vi "HiSPARCIII.vi"(6 "Files in":T1, 8 "Status/Errors in":refnum<vi>, 9 "Mode in":T2={"Mode"=enum."Dialog", "Expert?"=FALSE, "Dialog?"=FALSE}, 10 "Control Parameters [] in":T3[](array[typedef]) {"Aux Byte Value" format="%02x"; "Max Real Value" format="%#_6e"; "Min Real Value" format="%#_6e"; "dReal/dByte" format="%#_6e"; "Byte Value" format="%02x"; "Identifier" format="%02x"}) -> (0 "Status/Errors out":refnum<vi>, 1 "Mode out":T2={"Mode"=enum."Dialog", "Expert?"=FALSE, "Dialog?"=FALSE}, 2 "Control Parameters [] out":T3[](array[typedef]) {"Aux Byte Value" format="%02x"; "Max Real Value" format="%#_6e"; "Min Real Value" format="%#_6e"; "dReal/dByte" format="%#_6e"; "Byte Value" format="%02x"; "Identifier" format="%02x"}, 4 "Files out":T1)   [LabVIEW 2010]
uses:
  Controls/Control_Parameters.ctl
  Controls/Master.ctl
  Controls/Mode.ctl
  Controls/Files.ctl
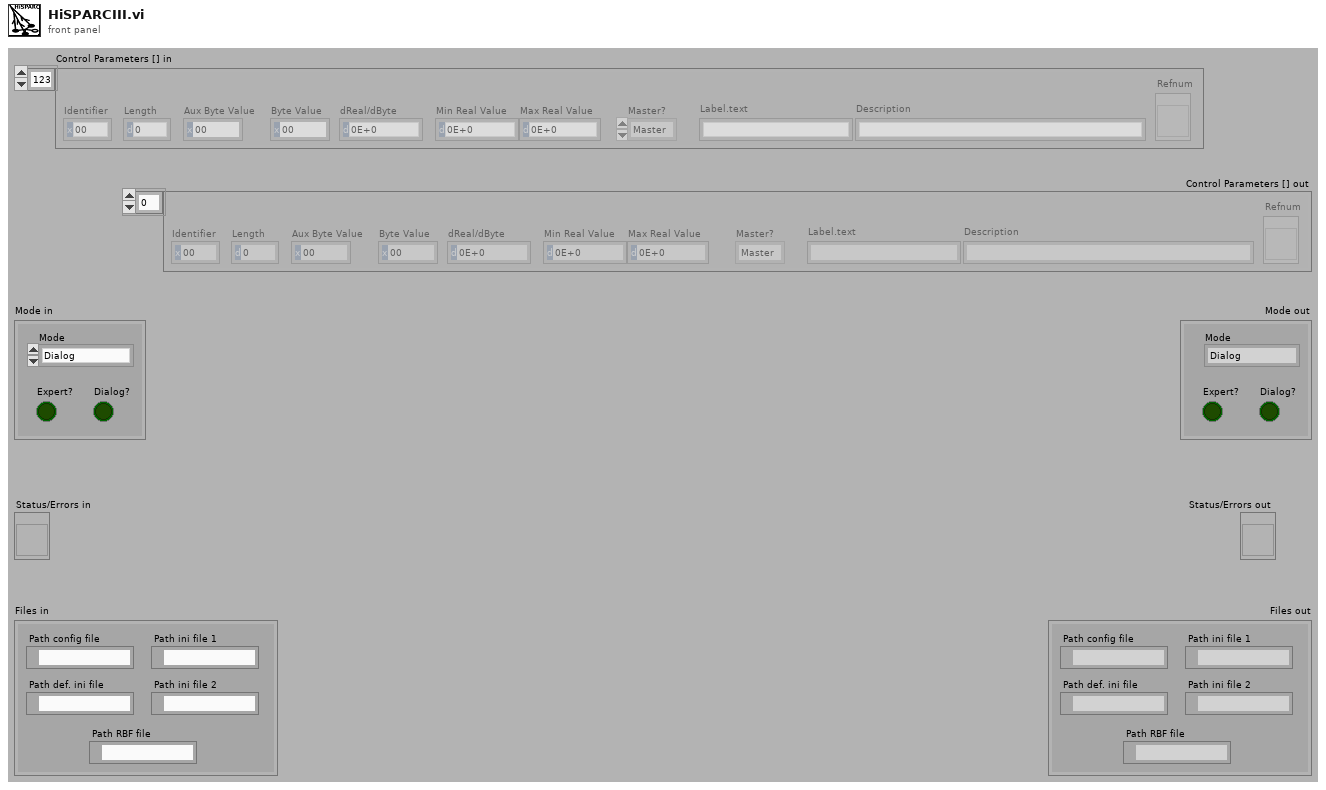
[diagram p1: front panel]
types:
  T1 = typedef "Files.ctl" = cluster{"Path config file":path, "Path def. ini file":path, "Path ini file 1":path, "Path ini file 2":path, "Path RBF file":path}
  T2 = typedef "Mode.ctl" = cluster{"Mode":enum8{"Stop", "Dialog", "Hisparc II", "Hisparc II DAQ", "Alignment"}, "Expert?":bool, "Dialog?":bool}
  T3 = typedef "Control_Parameters.ctl" = cluster{"Identifier":u8, "Length":u16, "Byte Value":u32, "dReal/dByte":dbl, "Min Real Value":dbl, "Max Real Value":dbl, "Master?":T4, "Label.text":string, "Description":string, "Refnum":refnum<vi>, "Aux Byte Value":u32}
  T4 = typedef "Master.ctl" = enum16{"Master", "Slave", "General"}
  T5 = enum8{"Stop", "Dialog", "Hisparc II", "Hisparc II DAQ", "Alignment"}
  T6 = typedef "Parameters.ctl" = cluster{"Mode":T2, "Stop loop":T7, "Send message":T8, "Write settings":T10, "Read bytes":T12, "Settings state":T13, "Button refs":T14, "Process messages":T15, "Data storage":T17, "Update screen":T22, "Alignment parameters":refnum<vi>, "Timer parameters":refnum<vi>, "Files":T1, "Status_id":refnum<vi>, "Time difference":refnum<vi>, "Satellites":refnum<vi>, "Calibration":T23, "Page Statistics 2":refnum<vi>, "Page Statistics":refnum<vi>}
  T7 = typedef "Stop_Loop.ctl" = cluster{"Settings changed?":bool, "Stop?":refnum<vi>}
  T8 = typedef "Send_Message.ctl" = cluster{"Send mode":T9, "Set parameter list":u8, "Get parameter list":u8, "Reset device":u8, "Length set settings message":i32, "Reset buttons?":bool, "Reset Master?":T4}
  T9 = typedef "Send_Message_Mode.ctl" = enum16{"Get parameters", "Set parameters", "From front panel", "From parameters", "Reset device", "Alignment"}
  T10 = typedef "Write_Settings.ctl" = cluster{"Options":T11}
  T11 = typedef "Write_Settings_Options.ctl" = enum16{"File 1", "File 2", "Alignment", "Reset"}
  T12 = typedef "Read_Bytes.ctl" = cluster{"Max bytes read":u32, "Max bytes reached?":bool}
  T13 = typedef "Settings_State.ctl" = cluster{"MAS locked?":refnum<vi>, "SLV locked?":refnum<vi>}
  T14 = typedef "Button_Refs.ctl" = cluster{"Stop program":refnum<vi>, "Save settings":refnum<vi>, "DAQ mode":refnum<vi>, "Reset settings":refnum<vi>, "Apply settings":refnum<vi>, "Reset MAS":refnum<vi>, "Reset SLV":refnum<vi>, "Local DBase?":refnum<vi>, "Last value DBase":bool, "Database":refnum<vi>, "Calibration":refnum<vi>, "Save settings 2":refnum<vi>}
  T15 = typedef "Process_Messages.ctl" = cluster{"Process message mode":T16, "Slave data?":bool, "Length get settings message":i32, "Delta time":dbl, "Data_Filter":cluster{"Filter_Data":bool, "Use_Thresh":bool, "Reduce data?":bool}, "Time_difference_stack":u64[], "Starting sec":u64, "Ending sec":u64, "Ending sec 2":u64, "MAS_Page_Thresh":refnum<vi>, "SLV_Page_Thresh":refnum<vi>, "Database":refnum<vi>}
  T16 = typedef "Process_Message_Mode.ctl" = enum16{"Error", "Measurement data", "Comparator data", "One Second"}
  T17 = typedef "Data_Storage.ctl" = cluster{"DB connection":T18, "Data storage condition":T20, "Detector number":u16, "# Messages to send":i32, "Database":refnum<vi>, "Password":string, "Last error message":cluster{"Last error message time stamp":T21, "Last error log":string, "Last error message":string}, "Status_id":refnum<vi>, "Hardware":enum8{"None", "HiSPARC I", "HiSPARC II", "HiSPARC III", "Unknown"}}
  T18 = typedef "DB_Connection.ctl" = cluster{"connection reference":T19, "Connected?":refnum<vi>, "ODBC Name":string}
  T19 = typedef "Conn ObjectReference.ctl" = refnum<k1>
  T20 = typedef "Data_Storage_Condition.ctl" = cluster{"Database?":bool}
  T21 = typedef "GPS_Timestamp.ctl" = cluster{"Seconds":u8, "Minutes":u8, "Hours":u8, "Day":u8, "Month":u8, "Year":u16}
  T22 = typedef "Update_Screen.ctl" = cluster{"Detector number":u16, "Hardware":enum8{"None", "HiSPARC I", "HiSPARC II", "HiSPARC III", "Unknown"}}
  T23 = typedef "Page_Calibration.ctl" = cluster{"GEN_Page_Calibrate":refnum<vi>, "MAS_Page_Gain":refnum<vi>, "MAS_Page_Offset":refnum<vi>, "SLV_Page_Gain":refnum<vi>, "SLV_Page_Offset":refnum<vi>, "MAS_Page_Common":refnum<vi>, "SLV_Page_Common":refnum<vi>}
  T24 = typedef "Devices.ctl" = cluster{"Master":refnum<vi>, "Slave":refnum<vi>}
  T25 = typedef "Queues.ctl" = cluster{"MAS":cluster{"Bytes":refnum<queue>, "Settings":refnum<queue>, "Errors":refnum<queue>, "Meas. data":refnum<queue>, "One Second":refnum<queue>, "Comp. data":refnum<queue>}, "SLV":cluster{"Bytes":refnum<queue>, "Settings":refnum<queue>, "Errors":refnum<queue>, "Meas. data":refnum<queue>, "One Second":refnum<queue>, "Comp. data":refnum<queue>}, "Events to store":refnum<queue>, "Events for screen":refnum<queue>, "One seconds MAS":refnum<queue>, "One seconds SLV":refnum<queue>, "Configuration message":refnum<queue>, "Comparator to store":refnum<queue>}
  T26 = typedef "Write_Data_Parameters.ctl" = cluster{"Stop loop":T7, "Data storage":T17}
  T27 = typedef "Process_Data_Parameters.ctl" = cluster{"Stop loop":T7, "Button refs":T14, "Process messages":T15, "Settings state":T13, "Mode":T2, "Alignment parameters":refnum<vi>, "Timer parameters":refnum<vi>, "Files":T1, "Time difference":refnum<vi>, "Alignment":T23, "Page Statistics":refnum<vi>}
  T28 = typedef "Main_Parameters.ctl" = cluster{"Mode":T2, "Stop loop":T7, "Send message":T8, "Write settings":T10, "Settings state":T13, "Button refs":T14, "Update screen":T22, "Files":T1, "DB connection":T18, "Status_id":refnum<vi>, "Time difference":refnum<vi>, "Satellites":refnum<vi>, "Alignment parameters":refnum<vi>, "Page Statistics 2":refnum<vi>, "Database":refnum<vi>, "Page Statistics":refnum<vi>}
  T29 = typedef "Read_Bytes_Parameters.ctl" = cluster{"Stop loop":T7, "Read bytes":T12}
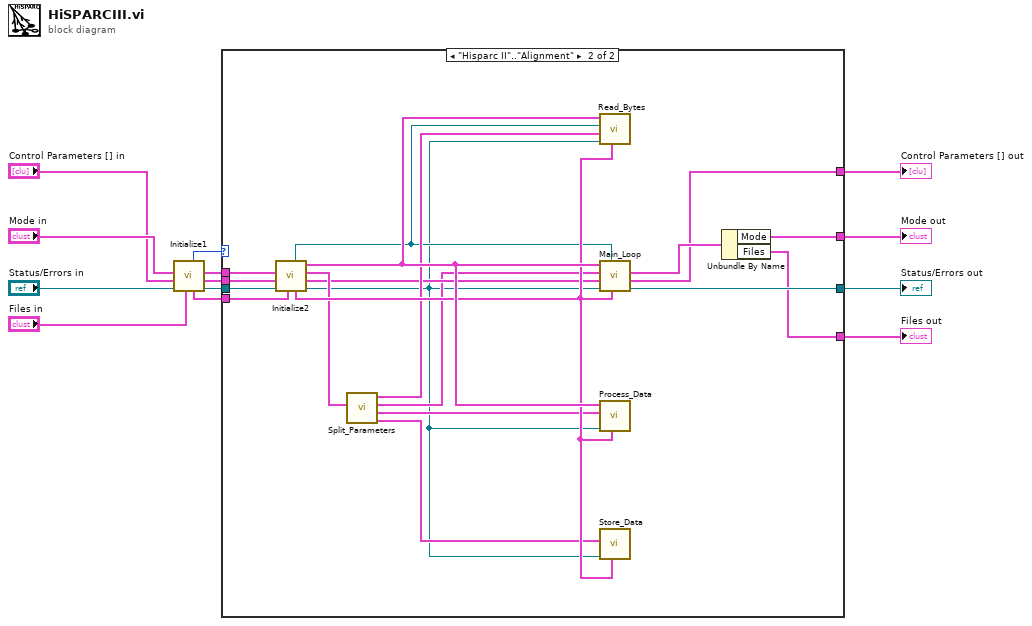
[diagram p0: block diagram]
diagram:
  n1 = call "Initialize1.vi"("Files in"="Files in", "Status/Errors in"="Status/Errors in", "Control Parameters [] in"="Control Parameters [] in", "Mode in"="Mode in") -> ("Status/Errors out"=w10:refnum<vi>, "Control Parameters [] out"=w4:T3[], "Mode out"=w6:T2, "Files out"=w7:T1, "Mode"=w5:T5)  [unwired: 3 out]
  n2 = case shown="\"Hisparc II\"..\"Alignment\"" w5 {
    tunnel: [w16 w32] -> w12
    tunnel: [w17 w30] -> w13
    tunnel: w4 -> [w17 w20]
    tunnel: w10 -> [w16 w36]
    tunnel: [w15 w31] -> w11
    tunnel: w6 -> [w15 w35]
    tunnel: w7 -> [w14 w19]
    tunnel: [w14 w18] -> w1
    frame Default {
    }
    frame "Hisparc II".."Alignment" {
      n3 = call "Initialize2.vi"("Files"=w19, "Status/Errors in"=w36, "Control Parameters [] in"=w20, "Mode"=w35) -> ("Status/Errors out"=w21:refnum<vi>, "Control Parameters [] out"=w24:T3[], "Parameters"=w28:T6, "Devices"=w34:T24, "Queues"=w29:T25, "Timer parameters out"=w23:refnum<vi>)  [unwired: 2 out]
      n4 = call "Split_Parameters.vi"("Parameters"=w28) -> ("Write data parameters"=w25:T26, "Process data parameters"=w26:T27, "Main parameters"=w22:T28, "Read bytes parameters"=w27:T29)  [unwired: 7 out]
      n5 = call "Read_Bytes.vi"("Queues"=w29, "Status/Errors in"=w21, "Read bytes parameters"=w27, "Timer parameters"=w23, "Devices"=w34) -> ()  [unwired: 7 out]
      n6 = call "Main_Loop.vi"("Queues"=w29, "Timer parameters"=w23, "Status/Errors in"=w21, "Control Parameters [] in"=w24, "Main parameters in"=w22, "Devices in"=w34) -> ("Status/Errors out"=w32:refnum<vi>, "Control Parameters [] out"=w30:T3[], "Main parameters out"=w33:T28)  [unwired: 3 out]
      n7 = call "Process_Data.vi"("Queues"=w29, "Status/Errors in"=w21, "Process data parameters in"=w26, "Devices in"=w34) -> ()  [unwired: 8 out]
      n8 = call "Store_Data.vi"("Queues"=w29, "Status/Errors in"=w21, "Write data parameters in"=w25) -> ()  [unwired: 1 in, 8 out]
      n9 = Unbundle By Name(w33) -> ("Mode"=w31:T2, "Files"=w18:T1)
    }
  }
  "Control Parameters [] out" <- w13
  "Status/Errors out" <- w12
  "Mode out" <- w11
  "Files out" <- w1
